vi "GUI_CH1_Comm_ZEROMQ_REQ.vi"() -> ()   [LabVIEW 2018]
uses:
  RxTx/RxTx.lvclass
  <vilib>/addons/zeromq/socket_type.ctl
  <vilib>/addons/zeromq/zmq_context.lvclass
  <vilib>/addons/zeromq/zeromq.lvlib
  <vilib>/addons/zeromq/zmq_socket.lvclass
panel:
  out "error out":errorcluster
  in  "stop":bool
  out "error out 3":errorcluster
  in  "RxTx.lvclass 2":refnum<class "RxTx.lvclass">
  # "Channel 1 - TCPIP Communication"
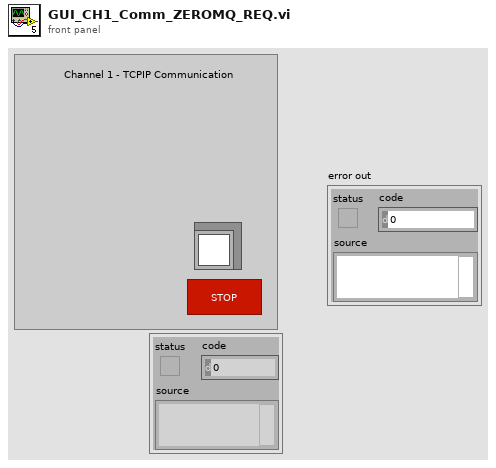
[diagram p1: front panel]
types:
  T1 = typedef "zeromq.lvlib/socket_type.ctl" = enum8{"ZMQ_PAIR", "ZMQ_PUB", "ZMQ_SUB", "ZMQ_REQ", "ZMQ_REP", "ZMQ_DEALER", "ZMQ_ROUTER", "ZMQ_PULL", "ZMQ_PUSH", "ZMQ_XPUB", "ZMQ_XSUB", "ZMQ_STREAM", "ZMQ_SERVER", "ZMQ_CLIENT", "ZMQ_RADIO", "ZMQ_DISH", "ZMQ_GATHER", "ZMQ_SCATTER", "ZMQ_DGRAM"}
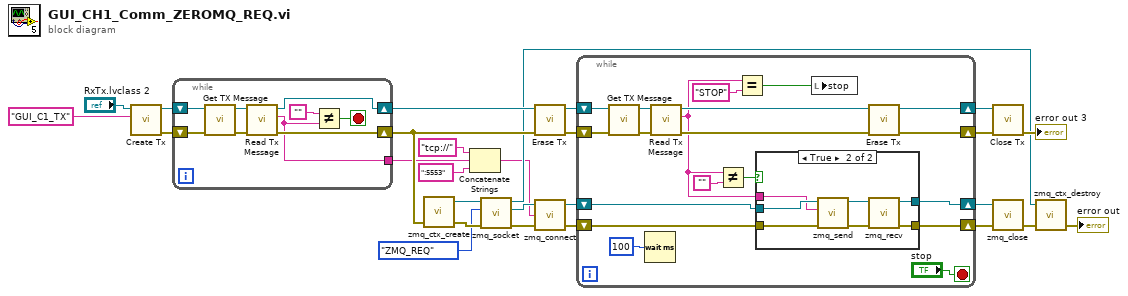
[diagram p0: block diagram]
diagram:
  n1 = call "Create Tx.vi"("Writer Name"="GUI_C1_TX", "RxTx in"="RxTx.lvclass 2") -> ("error out"=w19:errorcluster, "RxTx out"=w20:refnum<class "RxTx.lvclass">)  [unwired: 8 in]
  n2 = while {
    shift-right: [w32] -> w10
    shift-left: w19 -> [w31]
    shift-right: [w30] -> w23
    shift-left: w20 -> [w29]
    tunnel: [w28] -> w2
    stop <- w33 stop-if-true
    n3 = call "Get TX Message.vi"("error in (no error)"=w31, "RxTx in"=w29) -> ("error out"=w35:errorcluster, "RxTx out"=w36:refnum<class "RxTx.lvclass">)  [unwired: 8 in]
    n4 = call "Read Tx Message.vi"("error in (no error)"=w35, "RxTx in"=w36) -> ("error out"=w32:errorcluster, "Tx Message"=w28:string, "RxTx out"=w30:refnum<class "RxTx.lvclass">)  [unwired: 7 in]
    n5 = Not Equal?(x="", y=w28) -> (x != y?=w33:bool)
  }
  n6 = call <vilib>:"zmq_ctx_create.vi"("error in"=w10) -> ("error out"=w16:errorcluster, "context out"=w17:refnum<class "zmq_context.lvclass">)  [unwired: 3 in]
  n7 = Concatenate Strings("tcp://" ("endpoint"), w2, ":5553" ("endpoint")) -> (w4:string)
  n8 = call <vilib>:"zmq_socket.vi"("error in"=w16, "socket type"=socket_type."ZMQ_REQ", "context in"=w17) -> ("error out"=w3:errorcluster, "socket out"=w5:refnum<class "zmq_socket.lvclass">, "context out"=w9:refnum<class "zmq_context.lvclass">)  [unwired: 2 in]
  n9 = call "Erase Tx.vi"("error in (no error)"=w10, "RxTx in"=w23) -> ("error out"=w21:errorcluster, "RxTx out"=w22:refnum<class "RxTx.lvclass">)  [unwired: 8 in]
  n10 = call <vilib>:"zmq_connect.vi"("error in"=w3, "endpoint"=w4, "socket in"=w5) -> ("error out"=w7:errorcluster, "socket out"=w6:refnum<class "zmq_socket.lvclass">)  [unwired: 1 in]
  n11 = while {
    shift-right: [w55] -> w27
    shift-left: w22 -> [w48]
    shift-right: [w54] -> w26
    shift-left: w21 -> [w47]
    shift-right: [w42] -> w13
    shift-left: w7 -> [w43]
    shift-right: [w41] -> w12
    shift-left: w6 -> [w44]
    stop <- "stop" stop-if-true
    n12 = call "Get TX Message.vi"("error in (no error)"=w47, "RxTx in"=w48) -> ("error out"=w53:errorcluster, "RxTx out"=w49:refnum<class "RxTx.lvclass">)  [unwired: 8 in]
    n13 = Wait (ms)(milliseconds to wait=u32 100) -> ()  [unwired: 1 out]
    n14 = call "Read Tx Message.vi"("error in (no error)"=w53, "RxTx in"=w49) -> ("error out"=w50:errorcluster, "Tx Message"=w40:string, "RxTx out"=w51:refnum<class "RxTx.lvclass">)  [unwired: 7 in]
    n15 = Not Equal?(x=w40, y="") -> (x != y?=w37:bool)
    n16 = Equal?(x=w40, y="STOP" ("endpoint")) -> (x = y?=w38:bool)
    n17 = case shown="True" w37 {
      tunnel: w40 -> [_ w62]
      tunnel: w44 -> [w57 w64]
      tunnel: w43 -> [w56 w63]
      tunnel: [w56 w59] -> w42
      tunnel: [w57 w58] -> w41
      frame False {
      }
      frame True {
        n18 = call <vilib>:"zmq_send.vi"("error in"=w63, "data"=w62, "socket in"=w64) -> ("error out"=w60:errorcluster, "socket out"=w61:refnum<class "zmq_socket.lvclass">)  [unwired: 4 in]
        n19 = call <vilib>:"zmq_recv.vi"("error in"=w60, "socket in"=w61) -> ("error out"=w59:errorcluster, "socket out"=w58:refnum<class "zmq_socket.lvclass">)  [unwired: 3 in, 3 out]
      }
    }
    n20 = local write "stop"(w38) -> ()
    n21 = call "Erase Tx.vi"("error in (no error)"=w50, "RxTx in"=w51) -> ("error out"=w54:errorcluster, "RxTx out"=w55:refnum<class "RxTx.lvclass">)  [unwired: 8 in]
  }
  n22 = call "Close Tx.vi"("error in (no error)"=w26, "RxTx in"=w27) -> ("error out"=→"error out 3":errorcluster)  [unwired: 8 in, 1 out]
  n23 = call <vilib>:"zmq_close.vi"("error in"=w13, "socket"=w12) -> ("error out"=w14:errorcluster)  [unwired: 3 in]
  n24 = call <vilib>:"zmq_ctx_destroy.vi"("error in"=w14, "context in"=w9) -> ("error out"=→"error out":errorcluster)  [unwired: 3 in]
